vi "Image Distruction.vi"(8 "error in":errorcluster, 10 "Images":T1[](array[typedef])) -> (0 "error out":errorcluster)   [LabVIEW 2014]
uses:
  <vilib>/vision/Image Controls.llb/IMAQ Image.ctl
panel:
  # "LICENSED MATERIALS – PROPERTY OF IBM\nCopyright IBM Corp. 2016,\nALL RIGHTS RESERVED"
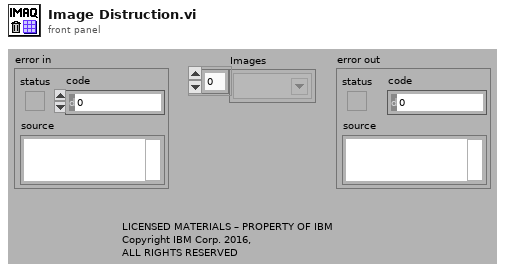
[diagram p1: front panel]
types:
  T1 = typedef "IMAQ Image.ctl" = refnum<image>
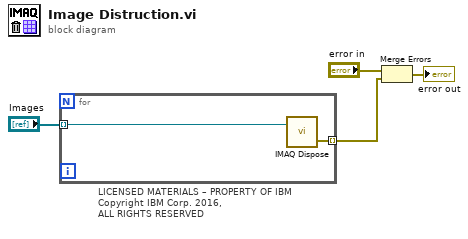
[diagram p0: block diagram]
diagram:
  # "LICENSED MATERIALS – PROPERTY OF IBM\nCopyright IBM Corp. 2016,\nALL RIGHTS RESERVED"
  n1 = for {
    tunnel: "Images" -> [w6] mode=indexing
    tunnel: [w5] -> w3 mode=indexing
    n2 = call "IMAQ Dispose"("Image"=w6) -> ("error out"=w5:errorcluster)  [unwired: 2 in, 3 out]
  }
  n3 = Merge Errors("error in", w3) -> (→"error out":errorcluster)
